vi "init.vi"() -> ()   [LabVIEW 2011]
uses:
  <vilib>/Rock Robotics/WPI/Camera/WPI_CameraImageSize.ctl
  <vilib>/Rock Robotics/WPI/Joystick/WPI_JoystickDeviceEnum.ctl
  <vilib>/Rock Robotics/SystemInterfaces/DIO/FPGA_DIOPWMChannel.ctl
  <vilib>/Rock Robotics/SystemInterfaces/Typedef/FPGA_TypedefDigitalModule.ctl
  <vilib>/Rock Robotics/SystemInterfaces/DIO/FPGA_DIOChannel.ctl
  <vilib>/Rock Robotics/WPI/Encoder/WPI_EncoderType.ctl
  <vilib>/Rock Robotics/SystemInterfaces/Typedef/FPGA_TypedefSolenoidModule.ctl
  <vilib>/Rock Robotics/WPI/Solenoid/WPI_SolenoidChannel.ctl
  <vilib>/Rock Robotics/SystemInterfaces/DIO/FPGA_DIORelayChannel.ctl
  <vilib>/Rock Robotics/WPI/SafetyOutput/WPI_SafetyOutputConfigMenu.ctl
  <vilib>/Rock Robotics/SystemInterfaces/AI/FPGA_AIChannel.ctl
  <vilib>/Rock Robotics/SystemInterfaces/Typedef/FPGA_TypedefAnalogModule.ctl
  <vilib>/Rock Robotics/WPI/MotorControl/WPI_MotorControlOpen Jaguar.vi
  <vilib>/Rock Robotics/WPI/Solenoid/WPI_SolenoidOpenSingle.vi
  <vilib>/Rock Robotics/WPI/RobotDrive/WPI_RobotDriveOpen4MotorWithJaguar.vi
  <vilib>/Rock Robotics/WPI/Compressor/WPI_CompressorGetSetRefNum.vi
  <vilib>/Rock Robotics/WPI/Camera/WPI_CameraWhite Balance Values.ctl
  <vilib>/Rock Robotics/WPI/Camera/WPI_CameraExposure Values.ctl
  <vilib>/Rock Robotics/WPI/Camera/WPI_CameraFrameRate.ctl
panel:
  in  "Image Size":T1=enum."160x120"
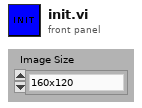
[diagram p1: front panel]
types:
  T1 = typedef "WPI_CameraImageSize.ctl" = enum16{"640x480", "320x240", "160x120"}
  T2 = typedef "FPGA_DIOPWMChannel.ctl" = enum8{"PWM 1", "PWM 2", "PWM 3", "PWM 4", "PWM 5", "PWM 6", "PWM 7", "PWM 8", "PWM 9", "PWM 10", "Invalid"}
  T3 = typedef "WPI_SafetyOutputConfigMenu.ctl" = enum16{"Enable", "Disable"}
  T4 = typedef "WPI_EncoderType.ctl" = enum16{"1x", "2x", "4x"}
  T5 = typedef "FPGA_DIOChannel.ctl" = enum8{"DIO 1", "DIO 2", "DIO 3", "DIO 4", "DIO 5", "DIO 6", "DIO 7", "DIO 8", "DIO 9", "DIO 10", "DIO 11", "DIO 12", "DIO 13", "DIO 14", "Invalid"}
  T6 = typedef "FPGA_DIORelayChannel.ctl" = enum8{"Relay 1", "Relay 2", "Relay 3", "Relay 4", "Relay 5", "Relay 6", "Relay 7", "Relay 8", "Invalid"}
  T7 = typedef "WPI_SolenoidChannel.ctl" = enum8{"Solenoid 1", "Solenoid 2", "Solenoid 3", "Solenoid 4", "Solenoid 5", "Solenoid 6", "Solenoid 7", "Solenoid 8", "Invalid"}
  T8 = typedef "FPGA_TypedefSolenoidModule.ctl" = enum16{"Solenoid Module 1", "Solenoid Module 2"}
  T9 = typedef "WPI_JoystickDeviceEnum.ctl" = enum16{"USB 1", "USB 2", "USB 3", "USB 4", "Kinect 1", "Kinect 2"}
  T10 = typedef "FPGA_TypedefDigitalModule.ctl" = enum16{"Digital Module 1", "Digital Module 2"}
  T11 = typedef "WPI_SolenoidDevRef.ctl" = cluster{"DevStatus":errorcluster, "Solenoid Module":T8, "Forward Solenoid Channel":T7, "Reverse Solenoid Channel":T7}
  T12 = typedef "WPI_DigitalInputDevRef.ctl" = cluster{"DevStatus":errorcluster, "DIO Channel":T5, "Digital Module":T10}
  T13 = typedef "WPI_CompressorDevRef.ctl" = cluster{"DevStatus":errorcluster, "DigitalInputDevRef":T12, "RelayDevRef":T14}
  T14 = typedef "WPI_RelayDevRef.ctl" = cluster{"DevStatus":errorcluster, "Relay Channel":T6, "Digital Module":T10, "Relay Direction":T15}
  T15 = typedef "WPI_RelayDirection.ctl" = enum16{"Both directions", "Forward only", "Reverse only"}
  T16 = typedef "FPGA_CounterEncoderSourceConvertionLVSourceType.ctl" = cluster{"DevStatus":errorcluster, "AnalogTriggerMode?":bool, "DigitalMode":cluster{"Digital Module":T10, "DIO Channel":T17}, "AnalogTriggerMode":cluster{"AnalogTriggerIndex":T18, "OutputType":T19}}
  T17 = typedef "FPGA_DIODigitalSourceChannel.ctl" = enum8{"DIO 1", "DIO 2", "DIO 3", "DIO 4", "DIO 5", "DIO 6", "DIO 7", "DIO 8", "DIO 9", "DIO 10", "DIO 11", "DIO 12", "DIO 13", "DIO 14", "Disabled"}
  T18 = typedef "FPGA_AnalogTriggerIndex.ctl" = enum8{"Trig 0", "Trig 1", "Trig 2", "Trig 3", "Trig 4", "Trig 5", "Trig 6", "Trig 7", "Invalid"}
  T19 = typedef "FPGA_AnalogTriggerOutType.ctl" = enum16{"InWindow", "TriggerState", "Rising", "Falling"}
  T20 = typedef "WPI_MotorControlDeviceRef.ctl" = cluster{"DeviceStatus":errorcluster, "Type":enum16{"PWM", "CAN"}, "PWM":cluster{"Digital Module":T10, "PWM Channel":T2, "DeadBand":T21}, "CAN":cluster{"Device Number":u8, "Control Mode":T22, "Semaphore":T23, "Max Vout":dbl}, "Invert":bool, "TransformRef":T24, "InvTransformRef":T24}
  T21 = typedef "WPI_PWMDeadband.ctl" = cluster{"Name":string, "maxPositivePwm":i32, "minPositivePwm":i32, "centerPwm":i32, "maxNegativePwm":i32, "minNegativePwm":i32, "angularRange":u16}
  T22 = typedef "WPI_CANJaguar_ControlMode.ctl" = enum8{"Percent VBus", "Current", "Speed", "Position", "Voltage"}
  T23 = typedef "Semaphore RefNum" = refnum<k1>
  T24 = typedef "WPI_PWMTransform_ConPane.ctl" = refnum<vi>
  T25 = typedef "WPI_JoystickDevRef.ctl" = cluster{"Device":T9}
  T26 = typedef "WPI_RobotDriveDevRef.ctl" = cluster{"DevStatus":errorcluster, "Motors[]":T20[], "Square Inputs":bool, "Max Output":dbl, "Isochronous":bool}
  T27 = typedef "WPI_EncoderDevRef.ctl" = cluster{"DevStatus":errorcluster, "EncoderIndex":T28, "CounterIndex":T29, "DistancePerCount":dbl, "Decoding Type":T4}
  T28 = typedef "FPGA_EncoderIdx.ctl" = enum8{"Enc 0", "Enc 1", "Enc 2", "Enc 3", "Invalid"}
  T29 = typedef "FPGA_CounterCtrSystemIndex.ctl" = enum8{"Ctr 0", "Ctr 1", "Ctr 2", "Ctr 3", "Ctr 4", "Ctr 5", "Ctr 6", "Ctr 7", "Invalid"}
  T30 = typedef "FPGA_AIChannel.ctl" = enum8{"AI 1", "AI 2", "AI 3", "AI 4", "AI 5", "AI 6", "AI 7", "AI 8", "Invalid"}
  T31 = typedef "FPGA_TypedefAnalogModule.ctl" = enum16{"Analog Module 1", "Analog Module 2"}
  T32 = typedef "WPI_AnalogChannelDevRef.ctl" = cluster{"DevStatus":errorcluster, "Analog Module":T31, "Analog Channel":T30}
  T33 = typedef "WPI_CameraFrameRate.ctl" = u32
  T34 = typedef "WPI_CameraExposure Values.ctl" = enum16{"Auto", "Flicker-free 50 Hz", "Flicker-free 60 Hz", "Hold current"}
  T35 = typedef "WPI_CameraWhite Balance Values.ctl" = enum16{"Auto", "Fixed indoor", "Fixed outdoor 1", "Fixed outdoor 2", "Fixed fluorescent 1", "Fixed fluorescent 2", "Hold current"}
  T36 = typedef "WPI_CameraDevRef.ctl" = cluster{"Camera Address":string, "CameraStatus":errorcluster, "Acquire Image Notifier":refnum<notifier>}
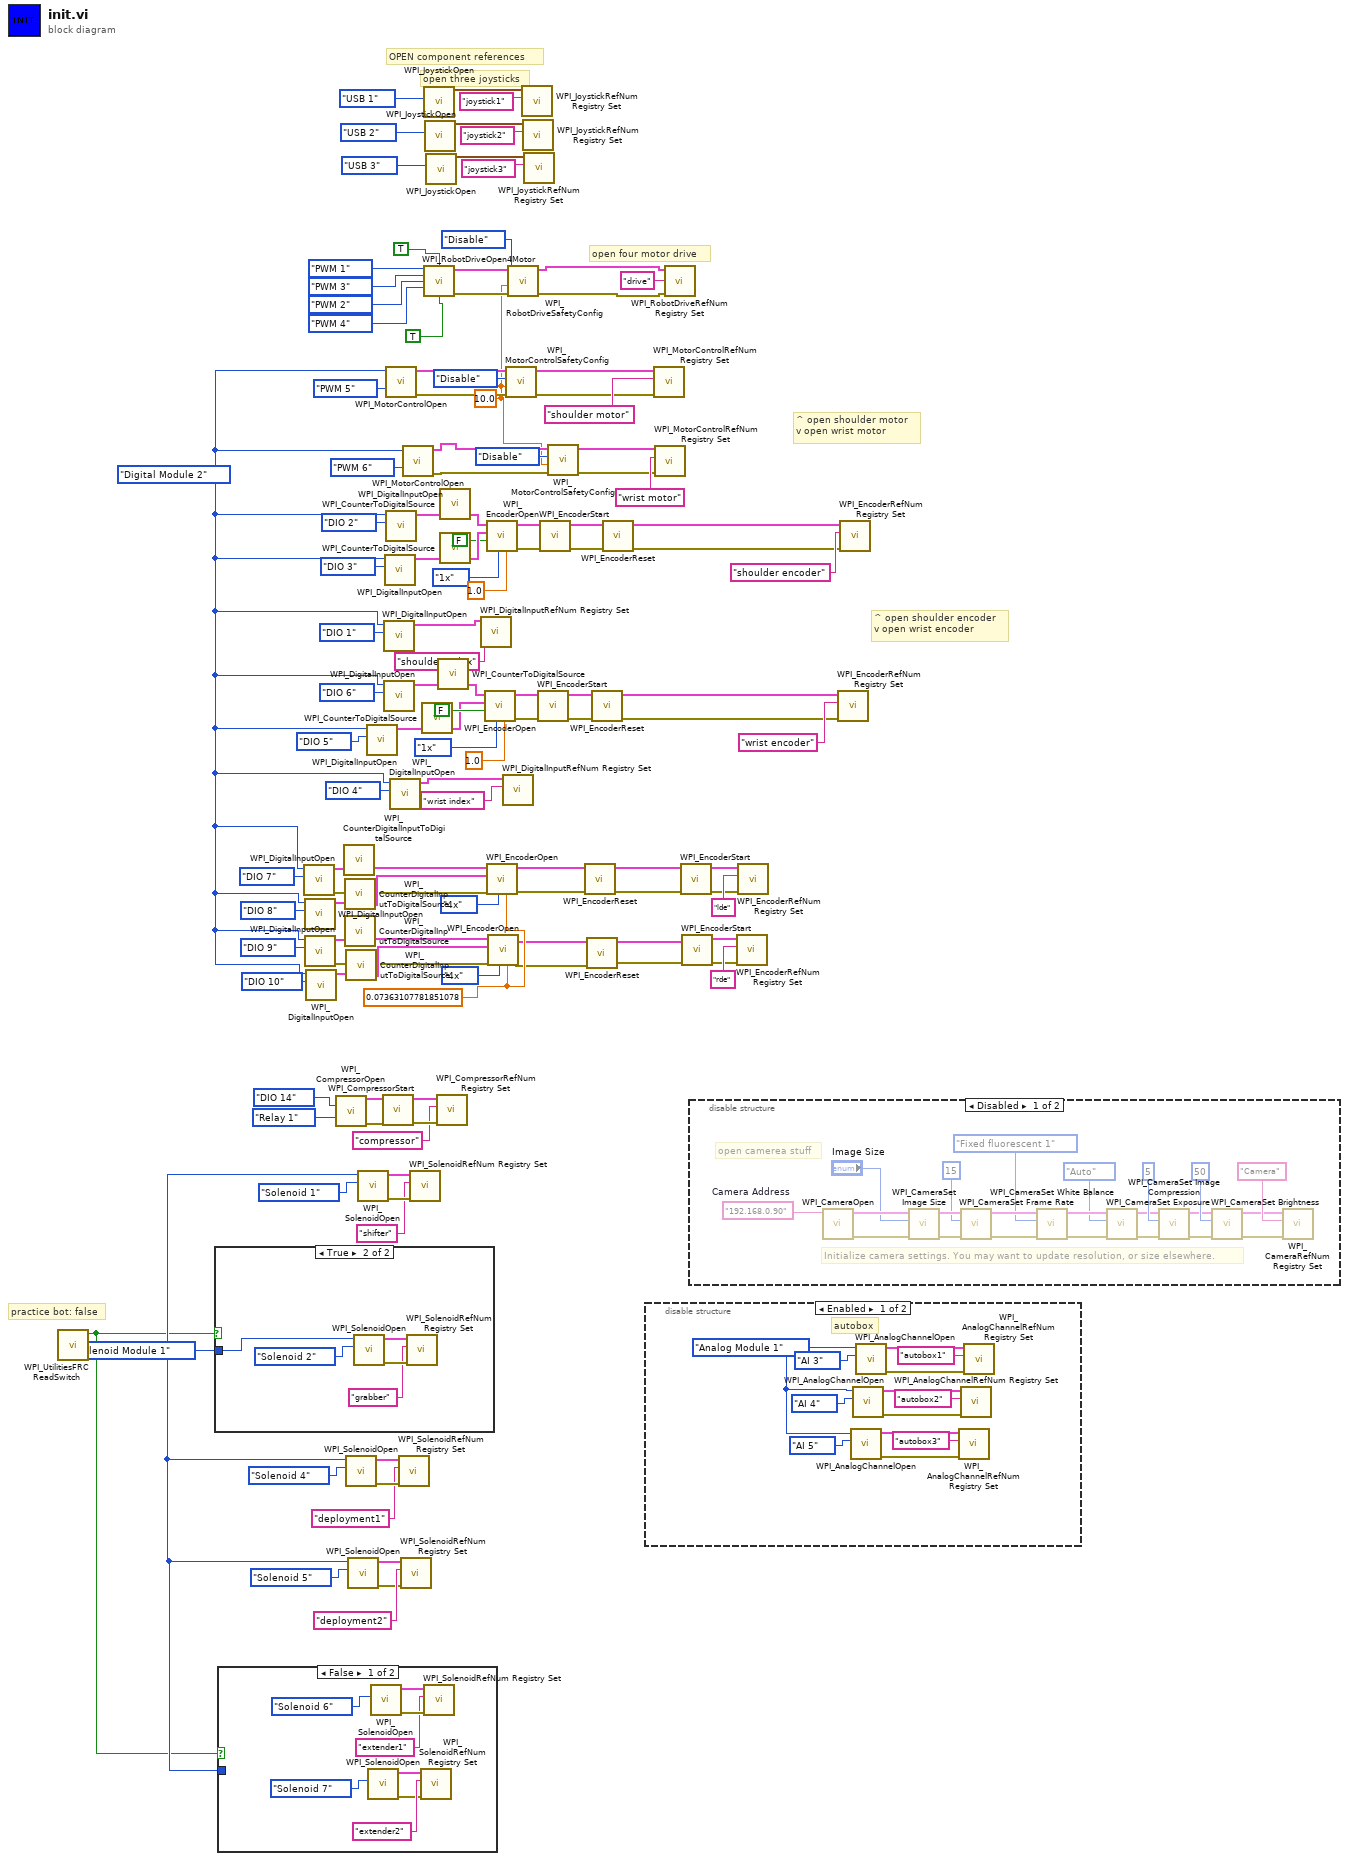
[diagram p0: block diagram]
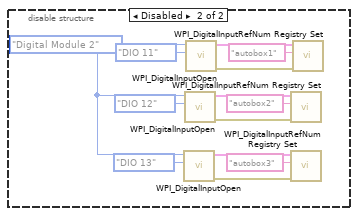
[diagram p2: hidden frame]
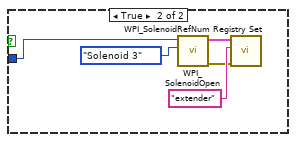
[diagram p3: hidden frame]
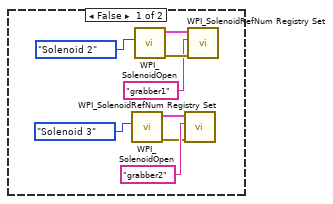
[diagram p4: hidden frame]
diagram:
  w4 = 10.0 ("timeout (s)")
  w57 = 0.07363107781851078 ("DistancePerCount")
  w58 = FPGA_TypedefSolenoidModule."Solenoid Module 1" ("Solenoid Module")
  w59 = FPGA_TypedefDigitalModule."Digital Module 2" ("DIO Module (Slot 4)")
  # "practice bot: false"
  # "^ open shoulder encoder\nv open wrist encoder"
  # "^ open shoulder motor\nv open wrist motor"
  # "open four motor drive"
  # "open three joysticks"
  # "OPEN component references"
  n1 = call <vilib>:"WPI_UtilitiesFRC ReadSwitch.vi"() -> ("switch state"=w1:bool)  [unwired: 1 in, 10 out]
  n2 = case shown="True" w1 {
    tunnel: w58 -> [_ w136]
    frame False {
      n3 = call-poly <vilib>:"WPI_SolenoidOpen.vi"("Solenoid Channel"=WPI_SolenoidChannel."Solenoid 3") -> ("error out"=w130:errorcluster, "SolenoidDevRef"=w131:T11)  [unwired: 2 in, 7 out]
      n4 = call-poly <vilib>:"WPI_SolenoidOpen.vi"("Solenoid Channel"=WPI_SolenoidChannel."Solenoid 2") -> ("error out"=w135:errorcluster, "SolenoidDevRef"=w134:T11)  [unwired: 2 in, 7 out]
      n5 = call <vilib>:"WPI_SolenoidRefNum Registry Set.vi"("error in (no error)"=w130, "refnum name"="grabber2", "SolenoidDevRef"=w131) -> ()  [unwired: 9 out]
      n6 = call <vilib>:"WPI_SolenoidRefNum Registry Set.vi"("error in (no error)"=w135, "refnum name"="grabber1", "SolenoidDevRef"=w134) -> ()  [unwired: 9 out]
    }
    frame True {
      n7 = call-poly <vilib>:"WPI_SolenoidOpen.vi"("Solenoid Channel"=WPI_SolenoidChannel."Solenoid 2", "Solenoid Module (Module 1)"=w136) -> ("error out"=w140:errorcluster, "SolenoidDevRef"=w139:T11)  [unwired: 1 in, 7 out]
      n8 = call <vilib>:"WPI_SolenoidRefNum Registry Set.vi"("error in (no error)"=w140, "refnum name"="grabber", "SolenoidDevRef"=w139) -> ()  [unwired: 9 out]
    }
  }
  n9 = case shown="False" w1 {
    tunnel: w58 -> [_ w149]
    frame False {
      n10 = call-poly <vilib>:"WPI_SolenoidOpen.vi"("Solenoid Channel"=WPI_SolenoidChannel."Solenoid 7") -> ("error out"=w143:errorcluster, "SolenoidDevRef"=w144:T11)  [unwired: 2 in, 7 out]
      n11 = call-poly <vilib>:"WPI_SolenoidOpen.vi"("Solenoid Channel"=WPI_SolenoidChannel."Solenoid 6") -> ("error out"=w148:errorcluster, "SolenoidDevRef"=w147:T11)  [unwired: 2 in, 7 out]
      n12 = call <vilib>:"WPI_SolenoidRefNum Registry Set.vi"("error in (no error)"=w143, "refnum name"="extender2", "SolenoidDevRef"=w144) -> ()  [unwired: 9 out]
      n13 = call <vilib>:"WPI_SolenoidRefNum Registry Set.vi"("error in (no error)"=w148, "refnum name"="extender1", "SolenoidDevRef"=w147) -> ()  [unwired: 9 out]
    }
    frame True {
      n14 = call-poly <vilib>:"WPI_SolenoidOpen.vi"("Solenoid Channel"=WPI_SolenoidChannel."Solenoid 3", "Solenoid Module (Module 1)"=w149) -> ("error out"=w151:errorcluster, "SolenoidDevRef"=w152:T11)  [unwired: 1 in, 7 out]
      n15 = call <vilib>:"WPI_SolenoidRefNum Registry Set.vi"("error in (no error)"=w151, "refnum name"="extender", "SolenoidDevRef"=w152) -> ()  [unwired: 9 out]
    }
  }
  n16 = call <vilib>:"WPI_DigitalInputOpen.vi"("DIO Channel"=FPGA_DIOChannel."DIO 7", "Digital Module (Module 1)"=w59) -> ("error out"=w31:errorcluster, "DigitalInputDevRef"=w42:T12)  [unwired: 1 in, 7 out]
  n17 = call <vilib>:"WPI_DigitalInputOpen.vi"("DIO Channel"=FPGA_DIOChannel."DIO 8", "Digital Module (Module 1)"=w59) -> ("DigitalInputDevRef"=w39:T12)  [unwired: 1 in, 8 out]
  n18 = call <vilib>:"WPI_DigitalInputOpen.vi"("DIO Channel"=FPGA_DIOChannel."DIO 9", "Digital Module (Module 1)"=w59) -> ("error out"=w30:errorcluster, "DigitalInputDevRef"=w33:T12)  [unwired: 1 in, 7 out]
  n19 = call <vilib>:"WPI_DigitalInputOpen.vi"("DIO Channel"=FPGA_DIOChannel."DIO 10", "Digital Module (Module 1)"=w59) -> ("DigitalInputDevRef"=w36:T12)  [unwired: 1 in, 8 out]
  n20 = call <vilib>:"WPI_CompressorOpen.vi"("Pressure Switch DIO Channel"=FPGA_DIOChannel."DIO 14", "Relay Channel"=FPGA_DIORelayChannel."Relay 1") -> ("CompressorDevRef"=w82:T13, "error out"=w83:errorcluster)  [unwired: 3 in, 9 out]
  n21 = call <vilib>:"WPI_CounterDigitalInputToDigitalSource.vi"("DigitalInputDevRef"=w42) -> ("Digital Source"=w43:T16)  [unwired: 6 out]
  n22 = call <vilib>:"WPI_CounterDigitalInputToDigitalSource.vi"("DigitalInputDevRef"=w39) -> ("Digital Source"=w38:T16)  [unwired: 6 out]
  n23 = call <vilib>:"WPI_CounterDigitalInputToDigitalSource.vi"("DigitalInputDevRef"=w33) -> ("Digital Source"=w32:T16)  [unwired: 6 out]
  n24 = call <vilib>:"WPI_CounterDigitalInputToDigitalSource.vi"("DigitalInputDevRef"=w36) -> ("Digital Source"=w37:T16)  [unwired: 6 out]
  n25 = call-poly <vilib>:"WPI_SolenoidOpen.vi"("Solenoid Channel"=WPI_SolenoidChannel."Solenoid 4", "Solenoid Module (Module 1)"=w58) -> ("error out"=w73:errorcluster, "SolenoidDevRef"=w72:T11)  [unwired: 1 in, 7 out]
  n26 = call-poly <vilib>:"WPI_SolenoidOpen.vi"("Solenoid Channel"=WPI_SolenoidChannel."Solenoid 5", "Solenoid Module (Module 1)"=w58) -> ("error out"=w68:errorcluster, "SolenoidDevRef"=w69:T11)  [unwired: 1 in, 7 out]
  n27 = call-poly <vilib>:"WPI_SolenoidOpen.vi"("Solenoid Channel"=WPI_SolenoidChannel."Solenoid 1", "Solenoid Module (Module 1)"=w58) -> ("error out"=w78:errorcluster, "SolenoidDevRef"=w77:T11)  [unwired: 1 in, 7 out]
  n28 = call <vilib>:"WPI_DigitalInputOpen.vi"("DIO Channel"=FPGA_DIOChannel."DIO 5", "Digital Module (Module 1)"=w59) -> ("DigitalInputDevRef"=w96:T12)  [unwired: 1 in, 8 out]
  n29 = call <vilib>:"WPI_CompressorStart.vi"("error in (no error)"=w83, "CompressorDevRef"=w82) -> ("error out"=w81:errorcluster, "CompressorDevRef"=w80:T13)  [unwired: 8 out]
  n30 = call <vilib>:"WPI_DigitalInputOpen.vi"("DIO Channel"=FPGA_DIOChannel."DIO 1", "Digital Module (Module 1)"=w59) -> ("DigitalInputDevRef"=w63:T12)  [unwired: 1 in, 8 out]
  n31 = call <vilib>:"WPI_DigitalInputOpen.vi"("DIO Channel"=FPGA_DIOChannel."DIO 6", "Digital Module (Module 1)"=w59) -> ("DigitalInputDevRef"=w95:T12)  [unwired: 1 in, 8 out]
  n32 = call <vilib>:"WPI_DigitalInputOpen.vi"("DIO Channel"=FPGA_DIOChannel."DIO 3", "Digital Module (Module 1)"=w59) -> ("DigitalInputDevRef"=w121:T12)  [unwired: 1 in, 8 out]
  n33 = call-poly <vilib>:"WPI_MotorControlOpen.vi"("PWM Channel"=FPGA_DIOPWMChannel."PWM 5", "Digital Module (Module 1)"=w59) -> ("error out"=w18:errorcluster, "MotorControlDeviceRef"=w19:T20)  [unwired: 5 in, 3 out]
  n34 = call <vilib>:"WPI_DigitalInputOpen.vi"("DIO Channel"=FPGA_DIOChannel."DIO 2", "Digital Module (Module 1)"=w59) -> ("DigitalInputDevRef"=w122:T12)  [unwired: 1 in, 8 out]
  n35 = call <vilib>:"WPI_DigitalInputOpen.vi"("DIO Channel"=FPGA_DIOChannel."DIO 4", "Digital Module (Module 1)"=w59) -> ("DigitalInputDevRef"=w60:T12)  [unwired: 1 in, 8 out]
  n36 = call <vilib>:"WPI_SolenoidRefNum Registry Set.vi"("error in (no error)"=w73, "refnum name"="deployment1", "SolenoidDevRef"=w72) -> ()  [unwired: 9 out]
  n37 = call <vilib>:"WPI_SolenoidRefNum Registry Set.vi"("error in (no error)"=w68, "refnum name"="deployment2", "SolenoidDevRef"=w69) -> ()  [unwired: 9 out]
  n38 = call-poly <vilib>:"WPI_MotorControlOpen.vi"("PWM Channel"=FPGA_DIOPWMChannel."PWM 6", "Digital Module (Module 1)"=w59) -> ("error out"=w12:errorcluster, "MotorControlDeviceRef"=w13:T20)  [unwired: 5 in, 3 out]
  n39 = call <vilib>:"WPI_SolenoidRefNum Registry Set.vi"("error in (no error)"=w78, "refnum name"="shifter", "SolenoidDevRef"=w77) -> ()  [unwired: 9 out]
  n40 = call-poly <vilib>:"WPI_CounterToDigitalSource.vi"("DigitalInputDevRef"=w96) -> ("Digital Source"=w97:T16)  [unwired: 6 out]
  n41 = call <vilib>:"WPI_JoystickOpen.vi"("JoystickDevice"=WPI_JoystickDeviceEnum."USB 1") -> ("JoystickDevRef"=w113:T25)  [unwired: 10 out]
  n42 = call-poly <vilib>:"WPI_RobotDriveOpen4Motor.vi"("Rear Left Motor"=FPGA_DIOPWMChannel."PWM 1", "Rear Right Motor Inverted"=TRUE, "Rear Right Motor"=FPGA_DIOPWMChannel."PWM 3" ("Rear Left Motor"), "Front Left Motor"=FPGA_DIOPWMChannel."PWM 2" ("Rear Left Motor"), "Front Right Motor"=FPGA_DIOPWMChannel."PWM 4" ("Rear Left Motor"), "Front Right Motor Inverted"=TRUE) -> ("RobotDriveDevRef"=w9:T26, "error out"=w8:errorcluster)  [unwired: 3 in, 5 out]
  n43 = call <vilib>:"WPI_JoystickOpen.vi"("JoystickDevice"=WPI_JoystickDeviceEnum."USB 2") -> ("JoystickDevRef"=w110:T25)  [unwired: 10 out]
  n44 = call <vilib>:"WPI_JoystickOpen.vi"("JoystickDevice"=WPI_JoystickDeviceEnum."USB 3") -> ("JoystickDevRef"=w107:T25)  [unwired: 10 out]
  n45 = call <vilib>:"WPI_CompressorRefNum Registry Set.vi"("error in (no error)"=w81, "refnum name"="compressor", "CompressorDevRef"=w80) -> ()  [unwired: 9 out]
  n46 = call-poly <vilib>:"WPI_CounterToDigitalSource.vi"("DigitalInputDevRef"=w95) -> ("Digital Source"=w94:T16)  [unwired: 6 out]
  n47 = call-poly <vilib>:"WPI_CounterToDigitalSource.vi"("DigitalInputDevRef"=w122) -> ("Digital Source"=w123:T16)  [unwired: 6 out]
  n48 = call-poly <vilib>:"WPI_CounterToDigitalSource.vi"("DigitalInputDevRef"=w121) -> ("Digital Source"=w120:T16)  [unwired: 6 out]
  n49 = call <vilib>:"WPI_DigitalInputRefNum Registry Set.vi"("refnum name"="shoulder index", "DigitalInputDevRef"=w63) -> ()  [unwired: 1 in, 9 out]
  n50 = call <vilib>:"WPI_EncoderOpen.vi"("DistancePerCount"=1.0, "Decoding Type"=WPI_EncoderType."1x", "Invert Direction (False)"=FALSE, "BSource"=w97, "ASource"=w94) -> ("error out"=w99:errorcluster, "EncoderDevRef"=w100:T27)  [unwired: 3 in, 2 out]
  n51 = call <vilib>:"WPI_EncoderOpen.vi"("DistancePerCount"=1.0, "Decoding Type"=WPI_EncoderType."1x", "Invert Direction (False)"=FALSE, "BSource"=w120, "ASource"=w123) -> ("error out"=w118:errorcluster, "EncoderDevRef"=w117:T27)  [unwired: 3 in, 2 out]
  n52 = call <vilib>:"WPI_EncoderOpen.vi"("DistancePerCount"=w57, "Decoding Type"=WPI_EncoderType."4x", "error in (no error)"=w31, "BSource"=w38, "ASource"=w43) -> ("error out"=w24:errorcluster, "EncoderDevRef"=w27:T27)  [unwired: 3 in, 2 out]
  n53 = call <vilib>:"WPI_EncoderOpen.vi"("DistancePerCount"=w57, "Decoding Type"=WPI_EncoderType."4x", "error in (no error)"=w30, "BSource"=w37, "ASource"=w32) -> ("error out"=w20:errorcluster, "EncoderDevRef"=w23:T27)  [unwired: 3 in, 2 out]
  n54 = call <vilib>:"WPI_DigitalInputRefNum Registry Set.vi"("refnum name"="wrist index", "DigitalInputDevRef"=w60) -> ()  [unwired: 1 in, 9 out]
  n55 = call <vilib>:"WPI_MotorControlSafetyConfig.vi"("error in (no error)"=w18, "timeout (s)"=w4, "mode"=WPI_SafetyOutputConfigMenu."Disable", "MotorControlDevRef"=w19) -> ("error out"=w17:errorcluster, "MotorControlDevRef"=w16:T20)  [unwired: 6 out]
  n56 = call <vilib>:"WPI_RobotDriveSafetyConfig.vi"("error in (no error)"=w8, "timeout (s)"=w4, "mode"=WPI_SafetyOutputConfigMenu."Disable", "RobotDriveDevRef"=w9) -> ("error out"=w6:errorcluster, "RobotDriveDevRef"=w7:T26)  [unwired: 6 out]
  n57 = call <vilib>:"WPI_JoystickRefNum Registry Set.vi"("refnum name"="joystick1", "JoystickDevRef"=w113) -> ()  [unwired: 1 in, 9 out]
  n58 = call <vilib>:"WPI_JoystickRefNum Registry Set.vi"("refnum name"="joystick2", "JoystickDevRef"=w110) -> ()  [unwired: 1 in, 9 out]
  n59 = call <vilib>:"WPI_JoystickRefNum Registry Set.vi"("refnum name"="joystick3", "JoystickDevRef"=w107) -> ()  [unwired: 1 in, 9 out]
  n60 = call <vilib>:"WPI_EncoderStart.vi"("error in (no error)"=w99, "EncoderDevRef"=w100) -> ("error out"=w51:errorcluster, "EncoderDevRef"=w101:T27)  [unwired: 8 out]
  n61 = call <vilib>:"WPI_EncoderStart.vi"("error in (no error)"=w118, "EncoderDevRef"=w117) -> ("error out"=w54:errorcluster, "EncoderDevRef"=w116:T27)  [unwired: 8 out]
  n62 = call <vilib>:"WPI_MotorControlSafetyConfig.vi"("error in (no error)"=w12, "timeout (s)"=w4, "mode"=WPI_SafetyOutputConfigMenu."Disable", "MotorControlDevRef"=w13) -> ("error out"=w10:errorcluster, "MotorControlDevRef"=w11:T20)  [unwired: 6 out]
  n63 = call <vilib>:"WPI_EncoderReset.vi"("error in (no error)"=w24, "EncoderDevRef"=w27) -> ("error out"=w25:errorcluster, "EncoderDevRef"=w26:T27)  [unwired: 8 out]
  n64 = call <vilib>:"WPI_EncoderReset.vi"("error in (no error)"=w20, "EncoderDevRef"=w23) -> ("error out"=w21:errorcluster, "EncoderDevRef"=w22:T27)  [unwired: 8 out]
  n65 = call <vilib>:"WPI_EncoderReset.vi"("error in (no error)"=w51, "EncoderDevRef"=w101) -> ("error out"=w50:errorcluster, "EncoderDevRef"=w52:T27)  [unwired: 8 out]
  n66 = call <vilib>:"WPI_EncoderReset.vi"("error in (no error)"=w54, "EncoderDevRef"=w116) -> ("error out"=w53:errorcluster, "EncoderDevRef"=w55:T27)  [unwired: 8 out]
  n67 = disable-structure shown="Enabled" {
    frame Enabled {
      w154 = FPGA_TypedefAnalogModule."Analog Module 1" ("Analog Module (Slot 1)")
      # "autobox"
      n68 = call <vilib>:"WPI_AnalogChannelOpen.vi"("Analog Channel"=FPGA_AIChannel."AI 5", "Analog Module (Module 1)"=w154) -> ("error out"=w160:errorcluster, "AIDeviceRef"=w159:T32)  [unwired: 1 in, 7 out]
      n69 = call <vilib>:"WPI_AnalogChannelOpen.vi"("Analog Channel"=FPGA_AIChannel."AI 4", "Analog Module (Module 1)"=w154) -> ("error out"=w161:errorcluster, "AIDeviceRef"=w162:T32)  [unwired: 1 in, 7 out]
      n70 = call <vilib>:"WPI_AnalogChannelOpen.vi"("Analog Channel"=FPGA_AIChannel."AI 3", "Analog Module (Module 1)"=w154) -> ("error out"=w166:errorcluster, "AIDeviceRef"=w165:T32)  [unwired: 1 in, 7 out]
      n71 = call <vilib>:"WPI_AnalogChannelRefNum Registry Set.vi"("error in (no error)"=w160, "refnum name"="autobox3", "AIDeviceRef"=w159) -> ()  [unwired: 9 out]
      n72 = call <vilib>:"WPI_AnalogChannelRefNum Registry Set.vi"("error in (no error)"=w161, "refnum name"="autobox2", "AIDeviceRef"=w162) -> ()  [unwired: 9 out]
      n73 = call <vilib>:"WPI_AnalogChannelRefNum Registry Set.vi"("error in (no error)"=w166, "refnum name"="autobox1", "AIDeviceRef"=w165) -> ()  [unwired: 9 out]
    }
    frame Disabled {
      w179 = FPGA_TypedefDigitalModule."Digital Module 2" ("DIO Module (Slot 4)")
      n74 = call <vilib>:"WPI_DigitalInputOpen.vi"("DIO Channel"=FPGA_DIOChannel."DIO 13", "Digital Module (Module 1)"=w179) -> ("error out"=w171:errorcluster, "DigitalInputDevRef"=w170:T12)  [unwired: 1 in, 7 out]
      n75 = call <vilib>:"WPI_DigitalInputOpen.vi"("DIO Channel"=FPGA_DIOChannel."DIO 12", "Digital Module (Module 1)"=w179) -> ("error out"=w173:errorcluster, "DigitalInputDevRef"=w172:T12)  [unwired: 1 in, 7 out]
      n76 = call <vilib>:"WPI_DigitalInputOpen.vi"("DIO Channel"=FPGA_DIOChannel."DIO 11", "Digital Module (Module 1)"=w179) -> ("error out"=w175:errorcluster, "DigitalInputDevRef"=w174:T12)  [unwired: 1 in, 7 out]
      n77 = call <vilib>:"WPI_DigitalInputRefNum Registry Set.vi"("error in (no error)"=w173, "refnum name"="autobox2", "DigitalInputDevRef"=w172) -> ()  [unwired: 9 out]
      n78 = call <vilib>:"WPI_DigitalInputRefNum Registry Set.vi"("error in (no error)"=w171, "refnum name"="autobox3", "DigitalInputDevRef"=w170) -> ()  [unwired: 9 out]
      n79 = call <vilib>:"WPI_DigitalInputRefNum Registry Set.vi"("error in (no error)"=w175, "refnum name"="autobox1", "DigitalInputDevRef"=w174) -> ()  [unwired: 9 out]
    }
  }
  n80 = call <vilib>:"WPI_MotorControlRefNum Registry Set.vi"("error in (no error)"=w17, "refnum name"="shoulder motor", "MotorControlDevRef"=w16) -> ()  [unwired: 9 out]
  n81 = call <vilib>:"WPI_MotorControlRefNum Registry Set.vi"("error in (no error)"=w10, "refnum name"="wrist motor", "MotorControlDevRef"=w11) -> ()  [unwired: 9 out]
  n82 = call <vilib>:"WPI_RobotDriveRefNum Registry Set.vi"("error in (no error)"=w6, "refnum name"="drive", "RobotDriveDevRef"=w7) -> ()  [unwired: 9 out]
  n83 = call <vilib>:"WPI_EncoderStart.vi"("error in (no error)"=w25, "EncoderDevRef"=w26) -> ("error out"=w44:errorcluster, "EncoderDevRef"=w45:T27)  [unwired: 8 out]
  n84 = call <vilib>:"WPI_EncoderStart.vi"("error in (no error)"=w21, "EncoderDevRef"=w22) -> ("error out"=w46:errorcluster, "EncoderDevRef"=w47:T27)  [unwired: 8 out]
  n85 = disable-structure shown="Disabled" {
    frame Disabled {
      w201 = "192.168.0.90"  # Camera Address
      # "open camerea stuff"
      # "Initialize camera settings. You may want to update resolution, or size elsewhere."
      n86 = call <vilib>:"WPI_CameraOpen.vi"("Camera Address"=w201) -> ("error out"=w191:errorcluster, "CameraDevRef"=w192:T36)  [unwired: 1 in, 8 out]
      n87 = call <vilib>:"WPI_CameraSet Image Size.vi"("error in (no error)"=w191, "Image Size"="Image Size", "CameraDevRef"=w192) -> ("error out"=w190:errorcluster, "CameraDevRef Out"=w193:T36)  [unwired: 7 out]
      n88 = call <vilib>:"WPI_CameraSet Frame Rate.vi"("error in (no error)"=w190, "Frame Rate (fps)"=T33 15, "CameraDevRef"=w193) -> ("error out"=w189:errorcluster, "CameraDevRef Out"=w195:T36)  [unwired: 7 out]
      n89 = call <vilib>:"WPI_CameraSet White Balance.vi"("error in (no error)"=w189, "White Balance"=WPI_CameraWhite_Balance_Values."Fixed fluorescent 1", "CameraDevRef"=w195) -> ("error out"=w188:errorcluster, "CameraDevRef Out"=w194:T36)  [unwired: 7 out]
      n90 = call <vilib>:"WPI_CameraSet Exposure.vi"("error in (no error)"=w188, "Exposure"=WPI_CameraExposure_Values."Auto", "CameraDevRef"=w194) -> ("error out"=w187:errorcluster, "CameraDevRef Out"=w197:T36)  [unwired: 7 out]
      n91 = call <vilib>:"WPI_CameraSet Image Compression.vi"("error in (no error)"=w187, "Compression"=5, "CameraDevRef"=w197) -> ("error out"=w186:errorcluster, "CameraDevRef Out"=w196:T36)  [unwired: 7 out]
      n92 = call <vilib>:"WPI_CameraSet Brightness.vi"("error in (no error)"=w186, "Brightness"=50, "CameraDevRef"=w196) -> ("error out"=w184:errorcluster, "CameraDevRef Out"=w185:T36)  [unwired: 7 out]
      n93 = call <vilib>:"WPI_CameraRefNum Registry Set.vi"("error in (no error)"=w184, "refnum name"="Camera", "CameraDevRef"=w185) -> ()  [unwired: 9 out]
    }
    frame Enabled {
    }
  }
  n94 = call <vilib>:"WPI_EncoderRefNum Registry Set.vi"("error in (no error)"=w46, "refnum name"="rde", "EncoderDevRef"=w47) -> ()  [unwired: 9 out]
  n95 = call <vilib>:"WPI_EncoderRefNum Registry Set.vi"("error in (no error)"=w44, "refnum name"="lde", "EncoderDevRef"=w45) -> ()  [unwired: 9 out]
  n96 = call <vilib>:"WPI_EncoderRefNum Registry Set.vi"("error in (no error)"=w50, "refnum name"="wrist encoder", "EncoderDevRef"=w52) -> ()  [unwired: 9 out]
  n97 = call <vilib>:"WPI_EncoderRefNum Registry Set.vi"("error in (no error)"=w53, "refnum name"="shoulder encoder", "EncoderDevRef"=w55) -> ()  [unwired: 9 out]
